vi "Output Actor Hardware Monitor.vi"() -> ()   [LabVIEW 2015]
uses:
  Event Input/Event Input.lvclass/Event Input.ctl
  input/input.lvclass
  Result/result.lvclass/result.ctl
  Result/result.lvclass
  Event Input/Event Input.lvclass
panel:
  in  "Hardware To Watch":string[](array[string])
  in  "Hardware Actor States":i32(listbox)
  in  "Stop Button":bool
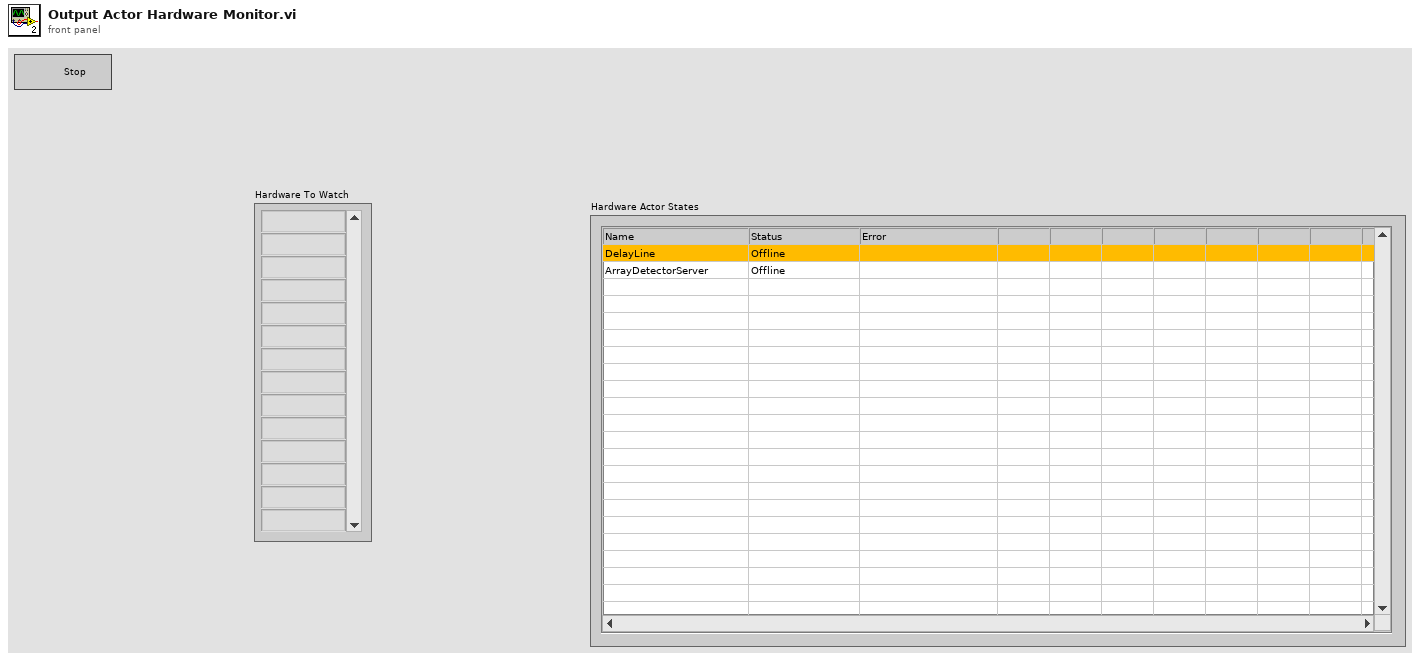
[diagram p1: front panel]
types:
  T1 = cluster{"input out":refnum<class "input.lvclass">, "Name":string, "Status":string, "error":errorcluster}
  T2 = cluster{"input out":refnum<class "input.lvclass">, "Name":string, "Status":string, "error out":errorcluster}
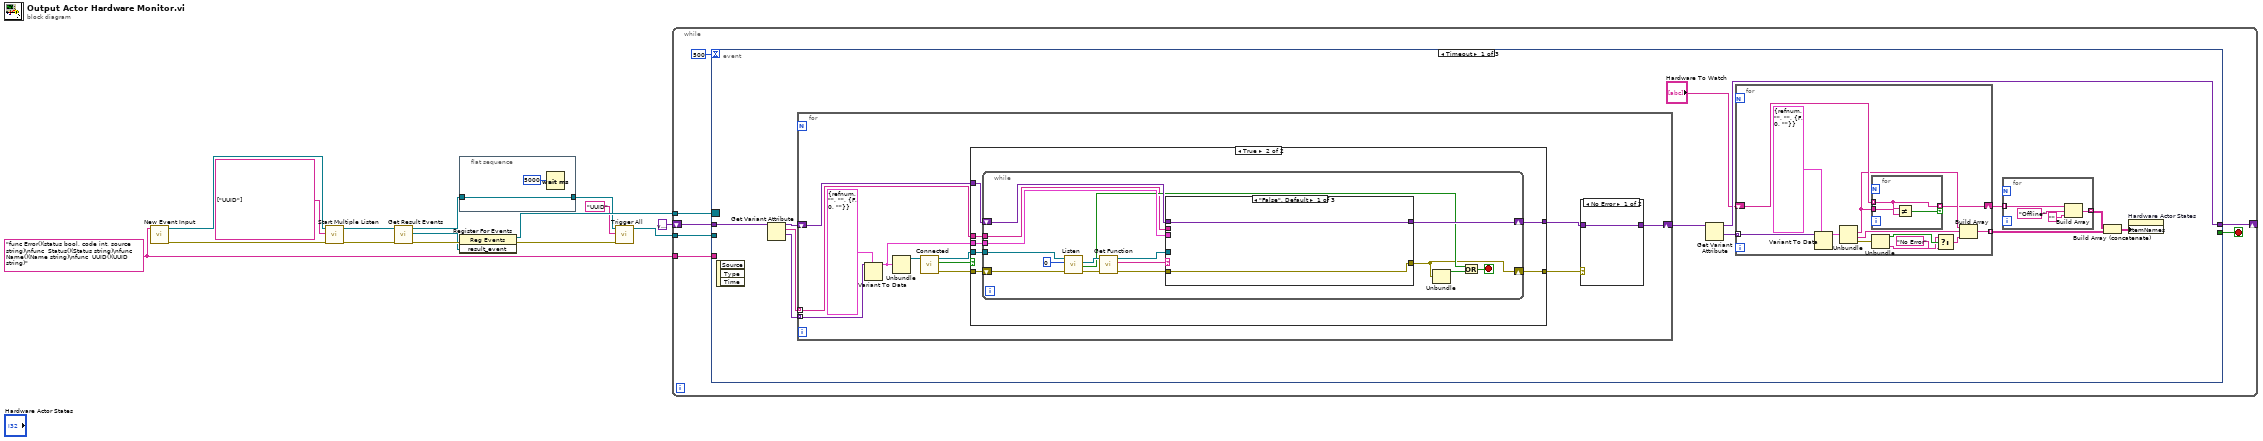
[diagram p0: block diagram]
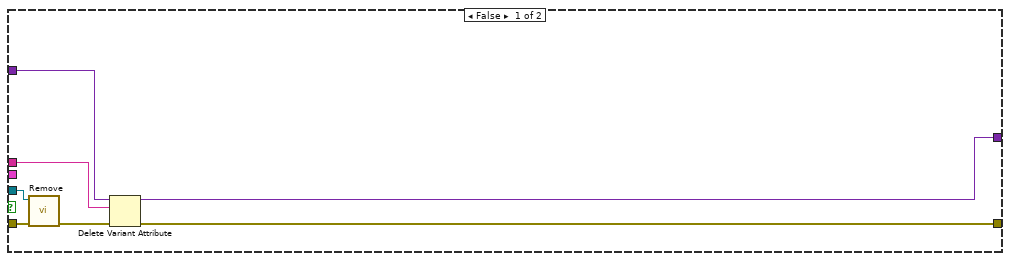
[diagram p2: hidden frame]
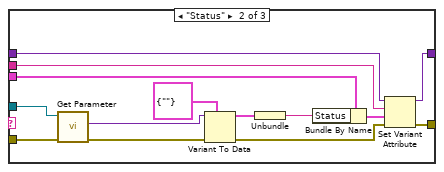
[diagram p3: hidden frame]
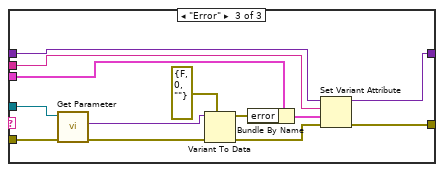
[diagram p4: hidden frame]
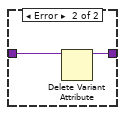
[diagram p5: hidden frame]
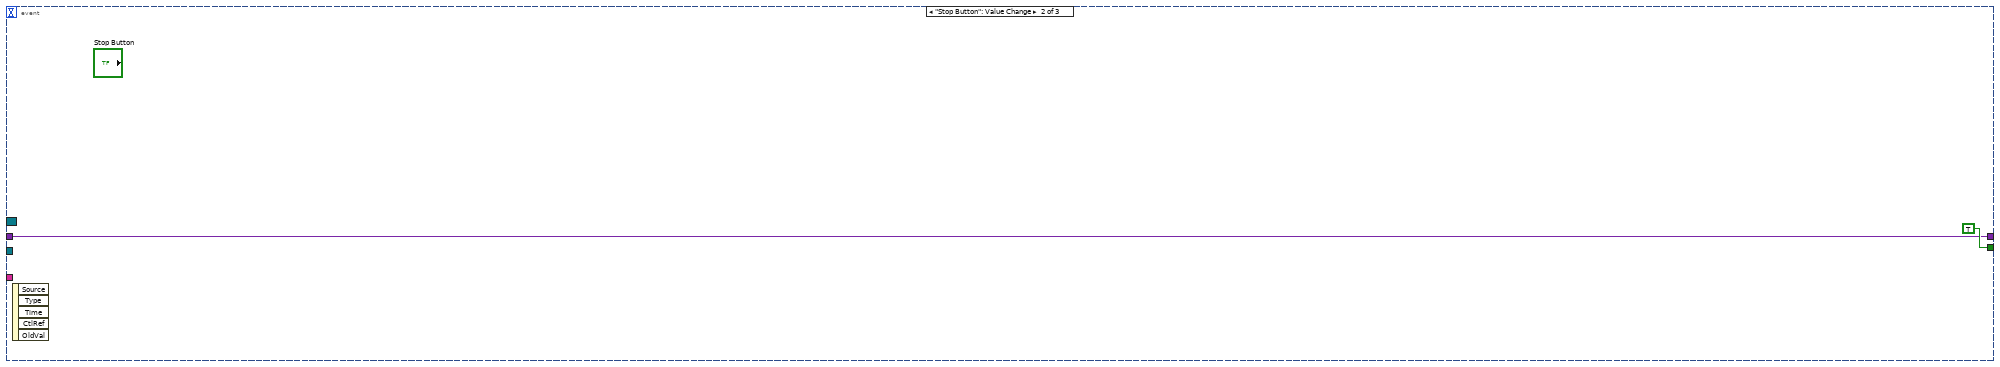
[diagram p6: hidden frame]
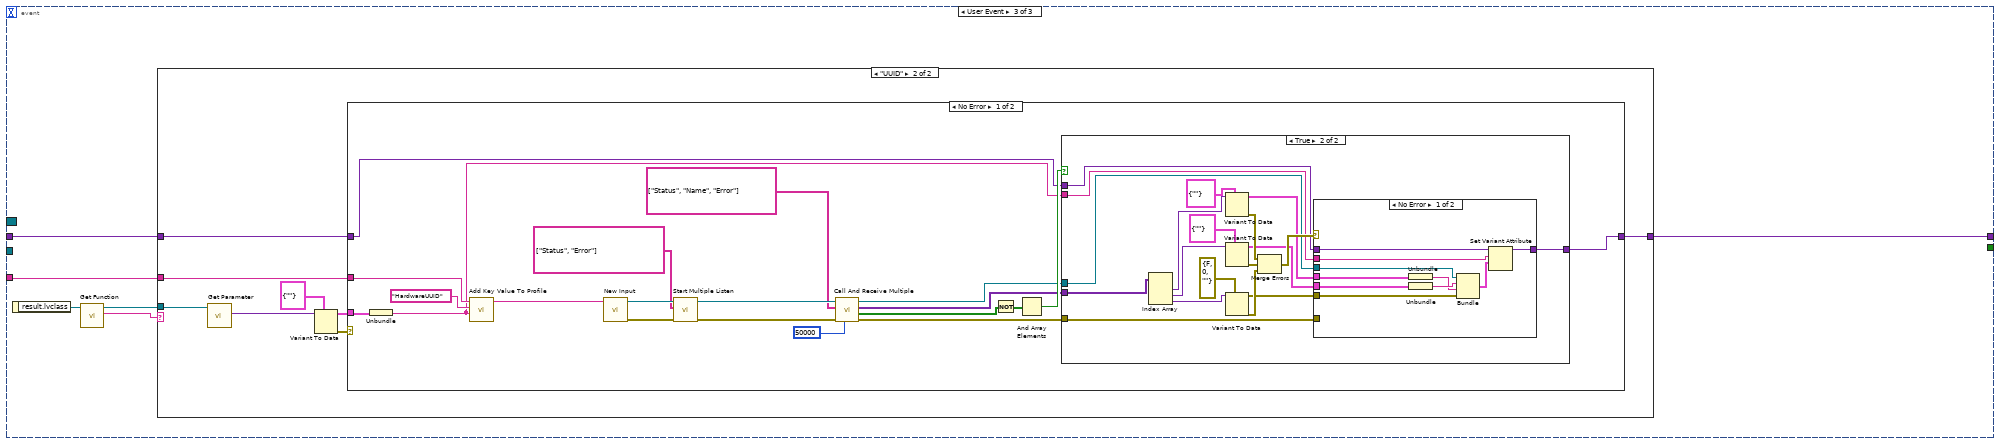
[diagram p7: hidden frame]
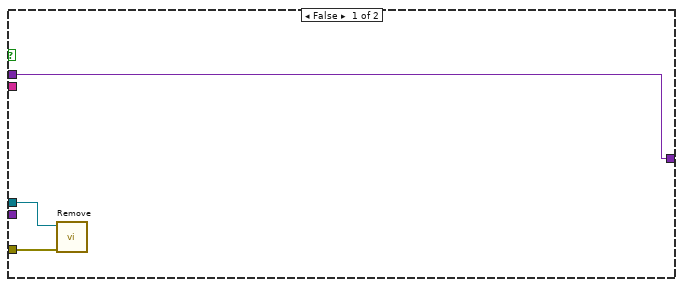
[diagram p9: hidden frame]
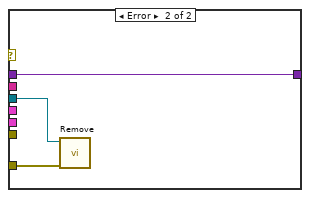
[diagram p10: hidden frame]
diagram:
  w7 = "func Error()(status bool, code int, source string)\nfunc  Status()(Status string)\nfunc  Name()(Name string)\nfunc  UUID()(UUID string)" ("Descriptor")
  n1 = call "New Event Input.vi"("Descriptor"=w7) -> ("error out"=w14:errorcluster, "event_input out"=w15:refnum<class "Event Input.lvclass">)  [unwired: 9 in]
  n2 = call "Start Multiple Listen.vi"("error in (no error)"=w14, "Functions"=string[] ["UUID"], "input in"=w15) -> ("error out"=w11:errorcluster, "input out"=w12:refnum<class "Event Input.lvclass">)  [unwired: 7 in]
  n3 = call "Get Result Events.vi"("error in (no error)"=w11, "event_input in"=w12) -> ("error out"=w10:errorcluster, "result_event"=w9:refnum<user-event>, "event_input out"=w5:refnum<class "Event Input.lvclass">)  [unwired: 7 in]
  n4 = flat-sequence {
    tunnel: [w17] -> w3
    tunnel: w5 -> [w17]
    frame #0 {
      n5 = Wait (ms)(milliseconds to wait=u32 5000) -> ()  [unwired: 1 out]
    }
  }
  n6 = register-events(error in=w10, w9) -> (reference out=w8:refnum<event-registration>, error out=w4:errorcluster)  [unwired: 1 in]
  n7 = call "Trigger All.vi"("error in (no error)"=w4, "Function"="UUID", "input in"=w3) -> ("input out"=w1:refnum<class "Event Input.lvclass">)  [unwired: 7 in, 1 out]
  n8 = while {
    tunnel: w8 -> [w23]
    tunnel: w1 -> [w22]
    tunnel: w7 -> [w21]
    shift-right: [w20] -> _
    shift-left: variant -> [w19]
    stop <- w24 stop-if-true
    n9 = event shown="[0] Timeout" {
      selector: w23 -> [_ _ _]
      dyn-events: _ -> [_ _ _]
      timeout: 500 -> [_ _ _]
      tunnel: [_ TRUE _] -> w24
      tunnel: w22 -> [_ _ _]
      tunnel: w21 -> [_ _ w135]
      tunnel: [w30 w131 w134] -> w20
      tunnel: w19 -> [w36 w131 w133]
      event Timeout {
        n10 = event-data() -> ()  [unwired: 1 in, 3 out]
        n11 = Get Variant Attribute(Variant=w36) -> (duplicate Variant=w34:variant, names=w33:string[], values=w35:variant[])  [unwired: 3 in, 1 out]
        n12 = for {
          tunnel: w35 -> [w67] mode=indexing
          shift-right: [w57] -> w32
          shift-left: w34 -> [w65]
          tunnel: w33 -> [w64] mode=indexing
          n13 = Variant To Data(type=T1 {"input out"=refnum, "Name"="", "Status"="", "error"={"status"=FALSE, "code"=0, "source"=""}} ("output cluster"), Variant=w67) -> (data=w61:T1)  [unwired: 1 in, 1 out]
          n14 = Unbundle(w61) -> ("input out"=w66:refnum<class "input.lvclass">)  [unwired: 3 out]
          n15 = call "Connected.vi"("input in"=w66) -> ("error out"=w60:errorcluster, "connected"=w63:bool, "input out"=w62:refnum<class "input.lvclass">)  [unwired: 8 in]
          n16 = case shown="True" w63 {
            tunnel: w62 -> [w75 w82]
            tunnel: w65 -> [w74 w80]
            tunnel: [w73 w77] -> w58
            tunnel: w64 -> [w72 w79]
            tunnel: w61 -> [_ w81]
            tunnel: w60 -> [w71 w78]
            tunnel: [w69 w76] -> w59
            frame False {
              n17 = call "Remove.vi"("error in (no error)"=w71, "input in"=w75) -> ("error out"=w70:errorcluster)  [unwired: 8 in, 1 out]
              n18 = Delete Variant Attribute(4:w70, 6:w72, 7:w74) -> (0:w69:errorcluster, 3:w73:variant)  [unwired: 1 out]
            }
            frame True {
              n19 = while {
                tunnel: w82 -> [w98]
                tunnel: w81 -> [w91]
                shift-right: [w89] -> w77
                shift-left: w80 -> [w90]
                tunnel: w79 -> [w83]
                shift-right: [w84] -> w76
                shift-left: w78 -> [w88]
                stop <- w86 stop-if-true
                n20 = call-dynamic "Listen.vi"("error in (no error)"=w88, "timeout in ms (-1)"=0, "input in"=w98) -> ("error out"=w93:errorcluster, "timed out?"=w87:bool, "result"=w96:refnum<class "result.lvclass">)  [unwired: 5 in, 1 out]
                n21 = call "Get Function.vi"("error in (no error)"=w93, "result in"=w96) -> ("error out"=w92:errorcluster, "function"=w95:string, "result out"=w94:refnum<class "result.lvclass">)  [unwired: 7 in]
                n22 = case shown="\"False\", Default" w95 {
                  tunnel: w94 -> [_ w113 w127]
                  tunnel: w92 -> [w99 w112 w126]
                  tunnel: w91 -> [_ w109 w123]
                  tunnel: w90 -> [w100 w106 w122]
                  tunnel: [w100 w105 w121] -> w89
                  tunnel: w83 -> [_ w104 w120]
                  tunnel: [w99 w101 w115] -> w84
                  frame "False", Default {
                  }
                  frame "Status" {
                    n23 = call-dynamic "Get Parameter.vi"("error in (no error)"=w112, "result in"=w113) -> ("error out"=w111:errorcluster, "Data"=w110:variant)  [unwired: 7 in, 1 out]
                    n24 = Variant To Data(error in=w111, type=cluster{"Status":string} {"Status"=""}, Variant=w110) -> (data=w108:cluster{"Status":string}, error out=w102:errorcluster)
                    n25 = Unbundle(w108) -> ("Status"=w107:string)
                    n26 = Bundle By Name(cluster=w109, "Status"=w107) -> (w103:T1)
                    n27 = Set Variant Attribute(Variant=w106, name=w104, value=w103, error in=w102) -> (Variant out=w105:variant, error out=w101:errorcluster)  [unwired: 1 out]
                  }
                  frame "Error" {
                    n28 = call-dynamic "Get Parameter.vi"("error in (no error)"=w126, "result in"=w127) -> ("error out"=w125:errorcluster, "Data"=w124:variant)  [unwired: 7 in, 1 out]
                    n29 = Variant To Data(error in=w125, type=errorcluster {"status"=FALSE, "code"=0, "source"=""} ("error out"), Variant=w124) -> (data=w117:errorcluster, error out=w116:errorcluster)
                    n30 = Bundle By Name(cluster=w123, "error"=w117) -> (w119:T1)
                    n31 = Set Variant Attribute(Variant=w122, name=w120, value=w119, error in=w116) -> (Variant out=w121:variant, error out=w115:errorcluster)  [unwired: 1 out]
                  }
                }
                n32 = Unbundle(w84) -> ("status"=w85:bool)  [unwired: 2 out]
                n33 = Or(x=w87, y=w85) -> (x .or. y?=w86:bool)
              }
            }
          }
          n34 = case shown="No Error" w59 {
            tunnel: w58 -> [w128 w130]
            tunnel: [w128 w129] -> w57
            frame No Error {
            }
            frame Error {
              n35 = Delete Variant Attribute(7:w130) -> (3:w129:variant)  [unwired: 2 in, 2 out]
            }
          }
        }
        n36 = Get Variant Attribute(Variant=w32) -> (duplicate Variant=w30:variant, values=w31:variant[])  [unwired: 3 in, 2 out]
        n37 = for {
          tunnel: w31 -> [w52] mode=indexing
          tunnel: [w44] -> w27 mode=indexing
          shift-right: [w41] -> w28
          shift-left: "Hardware To Watch" -> [w43]
          n38 = Variant To Data(type=T1 {"input out"=refnum, "Name"="", "Status"="", "error"={"status"=FALSE, "code"=0, "source"=""}} ("output cluster"), Variant=w52) -> (data=w51:T1)  [unwired: 1 in, 1 out]
          n39 = Unbundle(w51) -> ("Name"=w42:string, "Status"=w50:string, "error"=w49:errorcluster)  [unwired: 1 out]
          n40 = for {
            tunnel: w43 -> [w55] mode=indexing
            tunnel: w42 -> [w56]
            tunnel: [w55] -> w41 mode=indexing if=w54
            n41 = Not Equal?(x=w55, y=w56) -> (x != y?=w54:bool)
          }
          n42 = Unbundle(w49) -> ("status"=w48:bool, "source"=w47:string)  [unwired: 1 out]
          n43 = Select(t=w47, s=w48, f="No Error") -> (s? t:f=w45:string)
          n44 = Build Array(w42, w50, w45) -> (w44:string[])
        }
        n45 = for {
          tunnel: w28 -> [w40] mode=indexing
          tunnel: [w37] -> w26 mode=indexing
          n46 = Build Array(w40, "Offline" ("element"), "" ("element")) -> (w37:string[])
        }
        n47 = Build Array (concatenate)(w26, w27) -> (w25:string[][])
        n48 = property on="Hardware Actor States" class="MCListbox (strict)"("ItemNames"=w25) -> ()  [unwired: 2 in, 2 out]
      }
      event "Stop Button": Value Change {
        n49 = event-data() -> ()  [unwired: 1 in, 5 out]
      }
      event User Event {
        n50 = event-data() -> ("result.lvclass"=w138:refnum<class "result.lvclass">)  [unwired: 1 in]
        n51 = call "Get Function.vi"("result in"=w138) -> ("function"=w137:string, "result out"=w136:refnum<class "result.lvclass">)  [unwired: 8 in, 1 out]
        n52 = case shown="\"UUID\"" w137 {
          tunnel: w136 -> [_ w147]
          tunnel: w135 -> [_ w142]
          tunnel: [w139 w141] -> w134
          tunnel: w133 -> [w139 w140]
          frame Default {
          }
          frame "UUID" {
            n53 = call-dynamic "Get Parameter.vi"("result in"=w147) -> ("Data"=w146:variant)  [unwired: 8 in, 2 out]
            n54 = Variant To Data(type=cluster{"UUID":string} {"UUID"=""}, Variant=w146) -> (data=w144:cluster{"UUID":string}, error out=w143:errorcluster)  [unwired: 1 in]
            n55 = case shown="No Error" w143 {
              tunnel: w144 -> [w167 _]
              tunnel: w142 -> [w166 _]
              tunnel: [w149 w203] -> w141
              tunnel: w140 -> [w148 w203]
              frame No Error {
                n56 = Unbundle(w167) -> ("UUID"=w152:string)
                n57 = call "Add Key Value To Profile.vi"("Value"=w152, "Key"="HardwareUUID", "Descriptor"=w166) -> ("Flavoured Descriptor"=w164:string)  [unwired: 8 in]
                n58 = call "New Input.vi"("Descriptor"=w164) -> ("error out"=w161:errorcluster, "input out"=w163:refnum<class "input.lvclass">)  [unwired: 9 in]
                n59 = call "Start Multiple Listen.vi"("error in (no error)"=w161, "Functions"=string[] ["Status", "Error"], "input in"=w163) -> ("error out"=w159:errorcluster, "input out"=w160:refnum<class "input.lvclass">)  [unwired: 7 in]
                n60 = call "Call And Receive Multiple.vi"("timeout in ms (-1)"=50000, "error in (no error)"=w159, "Function"=string[] ["Status", "Name", "Error"] ("Functions"), "input in"=w160) -> ("error out"=w150:errorcluster, "timeout"=w156:bool[], "Data"=w153:variant[], "input out"=w151:refnum<class "input.lvclass">)  [unwired: 4 in]
                n61 = Not(x=w156) -> (.not. x?=w155:bool[])
                n62 = And Array Elements(Boolean array=w155) -> (logical AND=w154:bool)
                n63 = case shown="True" w154 {
                  tunnel: w153 -> [_ w189]
                  tunnel: w152 -> [_ w176]
                  tunnel: w151 -> [w170 w174]
                  tunnel: w150 -> [w169 w173]
                  tunnel: [w168 w172] -> w149
                  tunnel: w148 -> [w168 w171]
                  frame False {
                    n64 = call "Remove.vi"("error in (no error)"=w169, "input in"=w170) -> ()  [unwired: 8 in, 2 out]
                  }
                  frame True {
                    n65 = Index Array(array=w189) -> (element #1=w186:variant, element #2=w184:variant, element #3=w183:variant)  [unwired: 3 in]
                    n66 = Variant To Data(type=cluster{"Status":string} {"Status"=""}, Variant=w186) -> (data=w178:cluster{"Status":string}, error out=w182:errorcluster)  [unwired: 1 in]
                    n67 = Variant To Data(type=cluster{"Name":string} {"Name"=""}, Variant=w184) -> (data=w177:cluster{"Name":string}, error out=w181:errorcluster)  [unwired: 1 in]
                    n68 = Variant To Data(type=errorcluster {"status"=FALSE, "code"=0, "source"=""} ("error out"), Variant=w183) -> (data=w175:errorcluster, error out=w180:errorcluster)  [unwired: 1 in]
                    n69 = Merge Errors(w182, w181, w180) -> (w179:errorcluster)
                    n70 = case shown="No Error" w179 {
                      tunnel: w178 -> [w199 _]
                      tunnel: w177 -> [w198 _]
                      tunnel: w176 -> [w192 _]
                      tunnel: w175 -> [w195 _]
                      tunnel: w174 -> [w194 w202]
                      tunnel: w173 -> [_ w201]
                      tunnel: [w191 w200] -> w172
                      tunnel: w171 -> [w190 w200]
                      frame No Error {
                        n71 = Unbundle(w199) -> ("Status"=w196:string)
                        n72 = Unbundle(w198) -> ("Name"=w197:string)
                        n73 = Bundle("input out"=w194, "Name"=w197, "Status"=w196, "error out"=w195) -> (w193:T2)  [unwired: 1 in]
                        n74 = Set Variant Attribute(Variant=w190, name=w192, value=w193) -> (Variant out=w191:variant)  [unwired: 1 in, 2 out]
                      }
                      frame Error {
                        n75 = call "Remove.vi"("error in (no error)"=w201, "input in"=w202) -> ()  [unwired: 8 in, 2 out]
                      }
                    }
                  }
                }
              }
              frame Error {
              }
            }
          }
        }
      }
    }
  }
